vi "SLSC Convert Items - Min_Max to String.vi"(0 "minimum":string, 5 "maximum":string, 7 "min?":bool, 9 "max?":bool) -> (4 "minimum out":string, 6 "maximum out":string, 8 "minmax string":string)   [LabVIEW 2017, in "SLSC Tree Control.lvlib"]
doc: "Convert the min and max string values to the minmax string format used in the tree control."
uses:
  SLSC Tree Control.lvlib
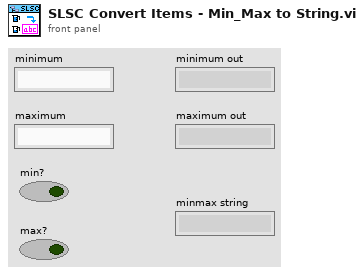
[diagram p1: front panel]
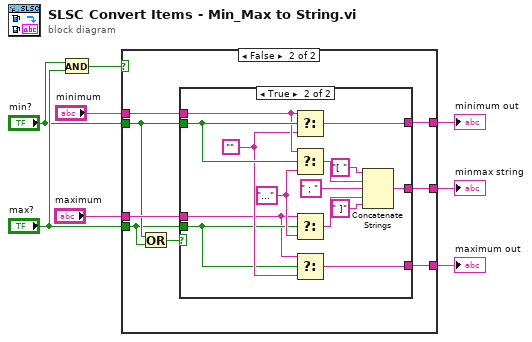
[diagram p0: block diagram]
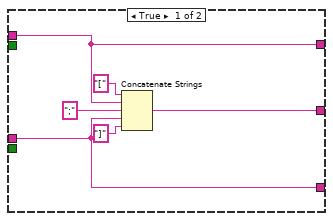
[diagram p2: hidden frame]
diagram:
  n1 = And(x="min?", y="max?") -> (x .and. y?=w8:bool)
  n2 = case shown="False" w8 {
    tunnel: [w14 w22] -> w5
    tunnel: "minimum" -> [w10 w21]
    tunnel: "maximum" -> [w9 w20]
    tunnel: "max?" -> [_ w17]
    tunnel: "min?" -> [_ w19]
    tunnel: [w10 w16] -> w2
    tunnel: [w9 w15] -> w1
    frame True {
      n3 = Concatenate Strings("[" ("string"), w10, ";" ("string"), w9, "]" ("string")) -> (w14:string)
    }
    frame False {
      n4 = Or(x=w19, y=w17) -> (x .or. y?=w18:bool)
      n5 = case shown="True" w18 {
        tunnel: [_ w36] -> w22
        tunnel: w21 -> [_ w27]
        tunnel: w20 -> [_ w24]
        tunnel: w19 -> [_ w28]
        tunnel: w17 -> [_ w25]
        tunnel: [_ w29] -> w16
        tunnel: [_ w23] -> w15
        frame False {
        }
        frame True {
          w26 = ""
          w34 = "..." ("f")
          n6 = Select(t=w27, s=w28, f=w26) -> (s? t:f=w29:string)
          n7 = Select(t=w27, s=w28, f=w34) -> (s? t:f=w32:string)
          n8 = Select(t=w24, s=w25, f=w34) -> (s? t:f=w31:string)
          n9 = Select(t=w24, s=w25, f=w26) -> (s? t:f=w23:string)
          n10 = Concatenate Strings("[ " ("string"), w32, " ; " ("string"), w31, " ]" ("string")) -> (w36:string)
        }
      }
    }
  }
  "minmax string" <- w5
  "maximum out" <- w1
  "minimum out" <- w2
